vi "tdms.parse.vi"() -> ()   [LabVIEW 2020, in "Nominal Client.lvclass"]
uses:
  Nominal Client.lvclass
  Nominal Client.lvclass/Nominal Client.ctl
  3e839d65-de1a-4bcc-af02-da9fc57c1e69.vi
  <vilib>/dlg_ctls.llb/Space Constant.vi
  private_data.set.vi
  <vilib>/Utility/file.llb/Application Directory.vi
  <vilib>/Utility/error.llb/Error Cluster From Error Code.vi
  submodules/reqwest-labview/lv-src/reqwest/create.vi
  ts.epochOfTimeUnit/build.epoch.vi
  ingest.trigger.vi
  catalog.wait_until_multiple_ingest_complete.vi
  <vilib>/addons/_JKI.lib/REST Client/classes/REST Client/REST Client.lvclass
  nominal types/workspace/workspace.lvclass
  submodules/reqwest-labview/lv-src/reqwest/reqwest.lvclass
  timestampMetadata/timestampMetadata.lvclass
  ts.epochOfTimeUnit/ts.epochOfTimeUnit.lvclass
panel:
  out "Created Dataset RIDs":string[](array[string])
  in  "File Path":path
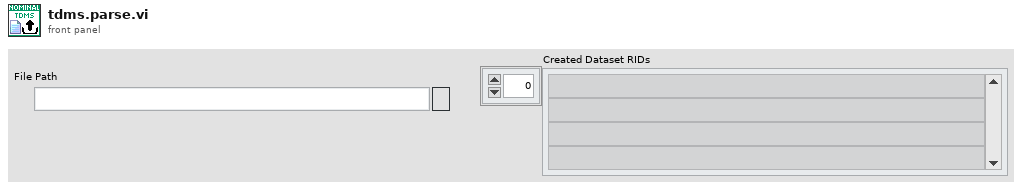
[diagram p1: front panel]
types:
  T1 = enum16{"open", "open or create", "create or replace", "create", "open (read-only)"}
  T2 = enum16{"DAYS", "HOURS", "MINUTES", "SECONDS", "MILLISECONDS", "MICROSECONDS", "NANOSECONDS", "PICOSECONDS"}
  T3 = cluster{"Properties":map{string, string}, "Labels":string[]}
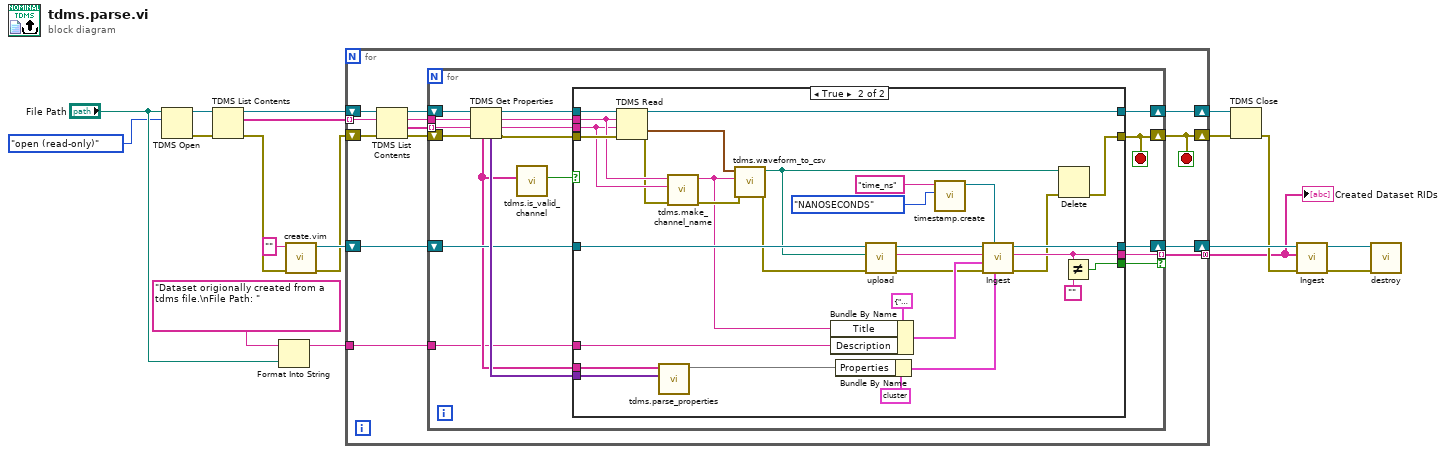
[diagram p0: block diagram]
diagram:
  n1 = TDMS Open(10:T1."open (read-only)" ("operation (0:open)"), 11:"File Path") -> (0:w18:errorcluster, 3:w19:refnum<k34>)  [unwired: 5 in]
  n2 = TDMS List Contents(4:w18, 7:w19) -> (0:w11:errorcluster, 2:w14:string[], 3:w17:refnum<k34>)  [unwired: 1 in, 1 out]
  n3 = Format Into String(initial string="Dataset origionally created from a tdms file.\nFile Path: ", "File Path") -> (resulting string=w2:string)  [unwired: 2 in, 1 out]
  n4 = call "create.vim"("error in"=w11, "API Token (string or path)"="") -> ("error out"=w10:errorcluster, "Nominal Client"=w13:refnum<class "Nominal Client.lvclass">)  [unwired: 8 in]
  n5 = for {
    shift-right: [w25] -> w15
    shift-left: w17 -> [w32]
    shift-right: [w20] -> w16
    shift-left: w10 -> [w31]
    tunnel: w14 -> [w30] mode=indexing
    shift-right: [w24] -> w9
    shift-left: w13 -> [w23]
    tunnel: [w22] -> w1 mode=concatenating
    tunnel: w2 -> [w21]
    stop <- w20 stop-if-true
    n6 = TDMS List Contents(4:w31, 6:w30, 7:w32) -> (0:w26:errorcluster, 1:w27:string[], 2:w28:string, 3:w29:refnum<k34>)
    n7 = for {
      tunnel: w28 -> [w47]
      tunnel: w27 -> [w46] mode=indexing
      shift-right: [w33] -> w20
      shift-left: w26 -> [w49]
      shift-right: [w43] -> w25
      shift-left: w29 -> [w50]
      shift-right: [w40] -> w24
      shift-left: w23 -> [w39]
      tunnel: [w36] -> w22 mode=indexing if=w35
      tunnel: w21 -> [w34]
      stop <- w33 stop-if-true
      n8 = TDMS Get Properties(8:w49, 9:w46, 10:w47, 11:w50) -> (0:w44:errorcluster, 1:w41:string, 2:w42:string, 3:w45:refnum<k34>, 4:w48:variant[], 6:w38:string[])  [unwired: 2 in]
      n9 = call "tdms.is_valid_channel.vi"("TDMS Property Names"=w38) -> ("Valid Channel"=w37:bool)  [unwired: 10 in]
      n10 = case shown="True" w37 {
        tunnel: w48 -> [_ w77]
        tunnel: w38 -> [_ w78]
        tunnel: w45 -> [w53 w85]
        tunnel: w44 -> [w52 w84]
        tunnel: [w53 w83] -> w43
        tunnel: [w52 w61] -> w33
        tunnel: w42 -> [_ w81]
        tunnel: w41 -> [_ w80]
        tunnel: [w51 w79] -> w40
        tunnel: w39 -> [w51 w75]
        tunnel: [_ w71] -> w36
        tunnel: [_ w70] -> w35
        tunnel: w34 -> [_ w66]
        frame False {
        }
        frame True {
          n11 = TDMS Read(0:w85, 5:w81, 7:w80, 11:w84) -> (4:w83:refnum<k34>, 10:w82:waveform(dbl), 15:w68:errorcluster)  [unwired: 4 in, 3 out]
          n12 = call "tdms.parse_properties.vi"("Property Values"=w77, "Property Names"=w78) -> ("Property Map"=w73:map{string, string})  [unwired: 9 in]
          n13 = call "tdms.make_channel_name.vi"("error in"=w68, "Channel Name"=w80, "Group Name"=w81) -> ("error out"=w76:errorcluster, "channel name"=w64:string)  [unwired: 7 in]
          n14 = call "tdms.waveform_to_csv.vi"("error in"=w76, "Formatted Channel Name"=w64, "Waveform"=w82) -> ("error out"=w67:errorcluster, "new csv filepath"=w63:path)  [unwired: 7 in]
          n15 = Bundle By Name(cluster=cluster{"Title":string, "Description":string} {"Title"="", "Description"=""} ("Title and Description"), "Title"=w64, "Description"=w66) -> (w65:cluster{"Title":string, "Description":string})
          n16 = Bundle By Name(cluster=T3 {"Properties"={}, "Labels"=[]} ("Properties and Labels"), "Properties"=w73) -> (w72:T3)
          n17 = call "upload.vi"("error in"=w67, "File"=w63, "Nominal Client in"=w75) -> ("error out"=w58:errorcluster, "Path to S3 File"=w59:string, "Nominal Client out"=w57:refnum<class "Nominal Client.lvclass">)  [unwired: 6 in]
          n18 = call-poly "timestamp.create.vi"("Time Unit"=T2."NANOSECONDS", "Time Series Name"="time_ns") -> ("Timestamp Metadata"=w56:refnum<class "timestampMetadata.lvclass">)  [unwired: 9 in]
          n19 = call-poly "Ingest.vi"("Properties and Labels"=w72, "Timestamp Metadata"=w56, "error in"=w58, "Title and Description"=w65, "S3 Path to File"=w59, "Nominal Client in"=w57) -> ("error out"=w62:errorcluster, "datasetRid"=w71:string, "Nominal Client out"=w79:refnum<class "Nominal Client.lvclass">)  [unwired: 1 in, 2 out]
          n20 = Delete(path (use dialog)=w63, error in=w62) -> (error out=w61:errorcluster)  [unwired: 3 in, 2 out]
          n21 = Not Equal?(x=w71, y="") -> (x != y?=w70:bool)
        }
      }
    }
  }
  "Created Dataset RIDs" <- w1
  n22 = TDMS Close(8:w16, 11:w15) -> (0:w8:errorcluster)  [unwired: 1 out]
  n23 = call-poly "Ingest.vi"("error in"=w8, "datasetRid"=w1, "Nominal Client"=w9) -> ("error out"=w7:errorcluster, "Nominal Client out"=w6:refnum<class "Nominal Client.lvclass">)  [unwired: 7 in]
  n24 = call "destroy.vi"("error in"=w7, "Nominal Client"=w6) -> ()  [unwired: 9 in, 1 out]
